vi "EventLog.File.Convert.vi"() -> ()   [LabVIEW 2015]
uses:
  EventLog.Event.ctl
  EventLog.EventLevel.ctl
  EventLog.EventSource.ctl
  Translator/Translator.Message.ctl
  Translator/Translator.Global.vi
panel:
  out "End of File?":bool
  out "size (in bytes)":i64
  out "size(s)":i32
  out "offset (in bytes)":i64
  out "Events out":T1[](array[typedef]) {"ts" format="%<%X\n%x>T"}
  in  "error in":errorcluster
  out "error out":errorcluster
  in  "file":path=path "D:/Maszup/TMS/WABCO/LASER MARKING/SOFTWARE/logs/events/Events-20161005.log"
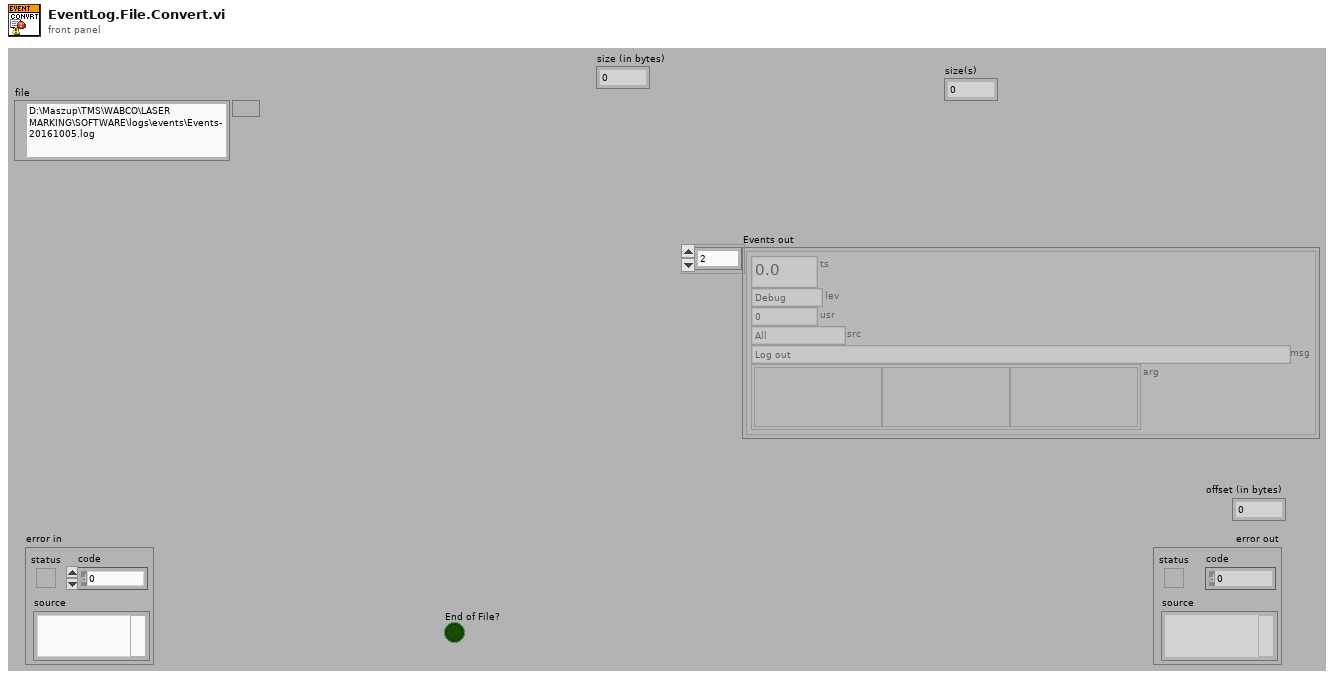
[diagram p1: front panel]
types:
  T1 = typedef "EventLog.Event.ctl" = cluster{"ts":dbl, "lev":T2, "usr":i32, "src":T3, "msg":T4, "arg":variant[]}
  T2 = typedef "EventLog.EventLevel.ctl" = enum8{"Debug", "Info", "Warning", "Error"}
  T3 = typedef "EventLog.EventSource.ctl" = enum16{"All", "Gui", "Ref", "File", "Arch", "Seq", "CPX", "Proda", "Laser", "Scan.P", "Scan.O"}
  T4 = typedef "Translator.Message.ctl" = enum16{"-", "Event confirmed", "Log out", "Log in", "Shutdown", "Cancel", "Start", "Begin time", "End time", "Duration", "Service Mode", "Ignore Results", "On", "Off", "OK", "NOK", "NOK %s", "Home", "Work", "Close", "Open", "In progress...", "Missing", "Empty", "Hardware failure", "Initial", "Out of range", "Error %d >> %s", "Error %d >> %s >> %s", "Msg %d >> %s", "Laser msg %d %s", "Laser cmd error %s %d", "Laser cmd failed %s", "Laser cmd warning %s", "Laser disconnected", "Laser status %s", "Laser already started", "Laser job unkonwn %s", "Laser job missing %s", "Laser job select failure %s", "Unable to start laser printing (%s)", "Unable to stop laser printing (%s)", "Laser marking aborted", "Unable to reset Laser Interlock (%s)", "Unable to trigger Laser. Laser not ready (%s)", "Laser job '%s' coordinates not configured", "Starting %s", "Quitting %s", "Configured", "Initializing", "Quitting", "Loading", "Running", "Stopped", "Summary", "Laser", "Do you want to continue?", "Press confirm button", "Station is not based. Do you want to exit?", "Station requires changeover. Do you want to run the test?", "Test options are not set as default. Do you want to continue?", "Product not detected. Do you want to continue?", "Product scan failed. Do you want to continue?", "Calibration", "Log out?", "System", "All", "IDLE", "Translating...%s", "Not found", "Alarm %s", "Run", "Skip", "Abort", "Repeat", "Please wait...", "Database disconnected", "Database disconnected - changeover disabled!", "Login to database successful", "Login to database failed: %d; %s", "Unable to check the product status of reference %d - database disconnected", "Unable to set the product status of reference %d - database disconnected", "Variant file backup %s", "Read steps (%s)", "Result", "Station armed!", "Station requires changeover!", "Select reference number...", "EMERGENCY BUTTON - press Control button", "EMERGENCY DOOR - press Control button", "Resetting Emergency...", "Unable to reset safety circuit - Emergency Button pressed", "Unable to reset safety circuit - Emergency Side Door open", "Station not based", "Station based", "Station not empty", "Station basing...", "No order", "Press Start to begin new order", "Scanning new order", "Order NOK. Correct or scan again", "Order OK. Press Accept", "Order ready", "Revolver incorrect", "Fork incorrect", "Revolver missing", "Revolver empty", "Container missing", "Offline results", "Door open", "Close the front door", "Press start button", "Done. Open the front door", "Running...", "Running...%.1f %%", "Pause", "Pause. NOK container missing", "Pause. OK container missing", "Pause. Revolver empty", "Pause. Revolver missing", "Pause. Revolver incorrect", "Pause. Fork missing", "Pause. Fork incorrect", "Pause. Too many failures", "Pause. One slot is not working", "Pause. Unable to move product to slot", "Pause. Unable to move back product pusher", "Pause. Unable to lift product", "Pause. Unable to move back product lifter", "Pause. Unable to move product arm to Work", "Pause. Unable to move product arm to NOK", "Pause. Unable to move product arm to OK", "Pause. Unable to unsuck the NOK product", "Pause. Unable to drop the NOK product", "Pause. Product OK missing", "Pause. Unable to unsuck the OK product", "Pause. Unable to drop the OK product", "Stopping...", "File '%s' is missing", "File '%s' is broken", "File '%s' is running", "Log file started (%s)", "Log file ended (%s)", "Log file ignored (%s)", "Log file exported (%s)", "Log file export failed (%s)", "Wrong serial number in log file", "Wrong reference number in log file", "Test steps are missing", "%s = %.3f", "Process param '%s' not found in DB", "Process param '%s' wrong order", "Process param '%s' value %.3f out of limits (%.3f; %.3f)", "Step%d param '%s' not found in DB", "Step%d param '%s' wrong order", "Step%d param '%s' value %.3f out of limits (%.3f; %.3f)", "Step%d EV '%s' not found in DB", "Step%d EV '%s' wrong order", "\"%s\" not found in DB", "\"%s\" wrong order", "\"%s\" value %.3f out of limits (%.3f; %.3f)", "\"%s\" not found in software", "Process init (%s)", "Process started", "Process restarted", "Process run", "Process done", "Process aborted", "Process aborted at work", "Process aborted at home", "Process error", "Process error at home", "Process error at work", "Process close", "Select plate from the order to process", "Do you want to start the process?", "Do you want to repeat the process?", "There is unfinished order. Do you want to put the new order?", "Product %s %d OK", "Product %s %d NOK", "Unable to unload the slot %s. Product missing in the slot", "Unable to unload the slot %s. Product already in the arm", "Unable to accept the product as OK. Product missing in slot %s", "Unable to accept the product as OK. Product could not drop into the container at slot %s", "Unable to accept the product as NOK. Product could not drop into the container at slot %s", "Scan failed. Error %s", "Scan failed. Scanner disconnected", "Scan failed. Wrong Wabco number %d, limit (%d,%d)", "Scan failed. Wrong serial number %d, limit (%d,%d)", "Scan failed. Wrong date %d, limit (%d,%d)", "Scan failed. Wrong product wabco number %d (expected %d)", "Scan failed. Wrong product serial number %d (expected > 0)", "Scan OK %s", "Scan failed. Unable to determine table position (%s)", "Scan failed. Timeout", "Tune failed. Scanner disconnected", "Tune failed. Timeout", "%s = %d", "%s = %d->%d", "Unable to set %s = %.2f - Air Pressure Inside off", "Unable to set digital output '%s' = %d", "Unable to activate air pressure inside - timeout", "Unable to activate air pressure inside - aborted", "Unable to switch on Air Main Valve - Air Pressure Inlet off", "Unable to switch on Air Main Valve - Door open", "Unable to switch off Air Main Valve - timeout", "Unable to switch off Air Main Valve - aborted", "Unable to rotate Table - timeout", "Unable to rotate Table - aborted", "Unable to rotate Table - Product Move not in Home position", "Unable to rotate Table - Air Pressure Inside off", "Unable to rotate Table - Product Lift A not in Home position", "Unable to rotate Table - Product Lift B not in Home position", "Unable to rotate Table - unlock before movement timeout", "Unable to rotate Table - lock after movement timeout", "Unable to move Table Lock to %s position - timeout", "Unable to move Table Lock to %s position - aborted", "Unable to move Table Lock to %s position - Air Pressure Inside off", "Unable to move Table Lock to %s position - Table not in position", "Unable to move Product Lift A to %s position - timeout", "Unable to move Product Lift B to %s position - timeout", "Unable to move Product Lift A to %s position - aborted", "Unable to move Product Lift B to %s position - aborted", "Unable to move Product Lift A to %s position - Air Pressure Inside off", "Unable to move Product Lift B to %s position - Air Pressure Inside off", "Unable to move Product Lift A to %s position - Table not locked", "Unable to move Product Lift B to %s position - Table not locked", "Unable to move Product Lift A to %s position - Product Arm not in Work position", "Unable to move Product Lift B to %s position - Product Arm not in Work position", "Unable to set Product Suction Gripper %s to %s - timeout", "Unable to set Product Suction Gripper %s to %s - aborted", "Unable to set Product Suction Gripper %s to %s - Air Pressure Inside off", "Unable to set Product Suction Gripper %s to %s - Table slot unkown", "Unable to move Product Arm to %s position - timeout", "Unable to move Product Arm to %s position - aborted", "Unable to move Product Arm to %s position - Air Pressure Inside off", "Unable to move Product Arm to %s position - Product Lift A not in Home position", "Unable to move Product Arm to %s position - Product Lift B not in Home position", "Unable to move Product to %s position - timeout", "Unable to move Product to %s position - aborted", "Unable to move Product to %s position - Air Pressure Inside off", "Unable to move Product to %s position - Table not in position"}
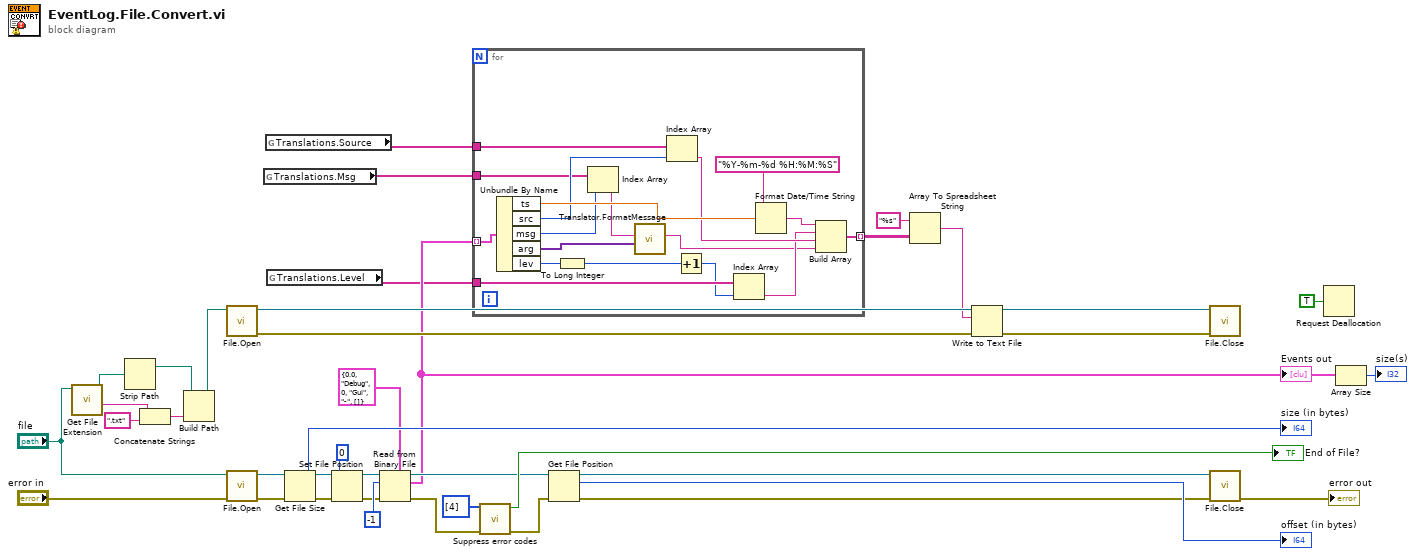
[diagram p0: block diagram]
diagram:
  n1 = call <vilib>:"Get File Extension.vi"("file"="file") -> ("filename without extension"=w17:string, "dup file"=w15:path)  [unwired: 6 in, 3 out]
  n2 = Strip Path(path=w15) -> (stripped path=w14:path)  [unwired: 1 out]
  n3 = Concatenate Strings(w17, ".txt" ("string")) -> (w13:string)
  n4 = Build Path(base path=w14, name or relative path=w13) -> (appended path=w12:path)
  n5 = call "File.Open.vi"("file"=w12) -> ("error out"=w11:errorcluster, "File ref out"=w9:refnum<file>)  [unwired: 9 in]
  n6 = call "File.Open.vi"("error in"="error in", "file"="file") -> ("error out"=w21:errorcluster, "File ref out"=w20:refnum<file>)  [unwired: 8 in]
  n7 = global read "Translator.Global.vi" "Translations.Msg"() -> (w4:string[])
  n8 = global read "Translator.Global.vi" "Translations.Source"() -> (w6:string[])
  n9 = global read "Translator.Global.vi" "Translations.Level"() -> (w5:string[])
  n10 = Get File Size(file=w20, error in=w21) -> (refnum out=w23:refnum<file>, size (in bytes)=→"size (in bytes)":i64, 0:w22:errorcluster)
  n11 = Set File Position(offset (in bytes) (0)=i64 0 ("read offset (in bytes)"), refnum=w23, error in=w22) -> (refnum out=w30:refnum<file>, error out=w31:errorcluster)  [unwired: 1 in]
  n12 = Read from Binary File(5:T1 {"ts"=0.0, "lev"=enum."Debug", "usr"=0, "src"=enum."Gui", "msg"=enum."-", "arg"=[]} ("element"), 8:w31, 10:-1 ("read count (ALL)"), 11:w30) -> (0:w26:errorcluster, 2:w7:T1[], 3:w29:refnum<file>)  [unwired: 2 in, 1 out]
  "Events out" <- w7
  n13 = for {
    tunnel: [w56] -> w3 mode=indexing
    tunnel: w7 -> [w55] mode=indexing
    tunnel: w5 -> [w53]
    tunnel: w6 -> [w44]
    tunnel: w4 -> [w43]
    n14 = Unbundle By Name(w55) -> ("ts"=w57:dbl, "src"=w49:T3, "msg"=w41:T4, "arg"=w46:variant[], "lev"=w52:T2)
    n15 = To Long Integer(number=w52) -> (32bit integer=w48:i32)
    n16 = Index Array(array=w43, index=w41) -> (element=w42:string)
    n17 = call "Translator.FormatMessage.vi"("Arguments"=w46, "Msg"=w42) -> ("Translated Msg"=w45:string)  [unwired: 9 in]
    n18 = Index Array(array=w44, index=w49) -> (element=w50:string)
    n19 = Increment(x=w48) -> (x+1=w51:i32)
    n20 = Index Array(array=w53, index=w51) -> (element=w47:string)
    n21 = Format Date/Time String(time format string (%c)="%Y-%m-%d %H:%M:%S", seconds (now)=w57) -> (date/time string=w54:string)  [unwired: 1 in]
    n22 = Build Array(w54, w47, w50, w45) -> (w56:string[])
  }
  n23 = call "Suppress error codes.vi"("error in (no error)"=w26, "suppress codes([43])"=i32[] [4]) -> ("error out"=w27:errorcluster, "suppressed"=→"End of File?":bool)  [unwired: 8 in]
  n24 = Get File Position(4:w27, 7:w29) -> (0:w24:errorcluster, 2:→"offset (in bytes)":i64, 3:w25:refnum<file>)
  n25 = Array To Spreadsheet String(array=w3, 3:"%s" ("format string")) -> (spreadsheet string=w1:string)  [unwired: 1 in]
  n26 = Write to Text File(file (use dialog)=w9, text=w1, error in=w11) -> (refnum out=w8:refnum<file>, error out=w10:errorcluster)  [unwired: 1 in, 1 out]
  n27 = call "File.Close.vi"("error in"=w10, "File ref in"=w8) -> ()  [unwired: 9 in, 1 out]
  n28 = call "File.Close.vi"("error in"=w24, "File ref in"=w25) -> ("error out"=→"error out":errorcluster)  [unwired: 9 in]
  n29 = Request Deallocation(TRUE ("flag")) -> ()
  n30 = Array Size(array=w7) -> (size(s)=→"size(s)":i32)
